vi "update tree.vi"(7 "status type":T1, 8 "error in (no error)":errorcluster, 10 "tag":string, 11 "TreeControl in":refnum<vi>) -> (0 "error out":errorcluster)   [LabVIEW 2016, in "FPGA Addon System Explorer.lvlib"]
uses:
  FPGA Addon System Explorer.lvlib
  reservation type.ctl
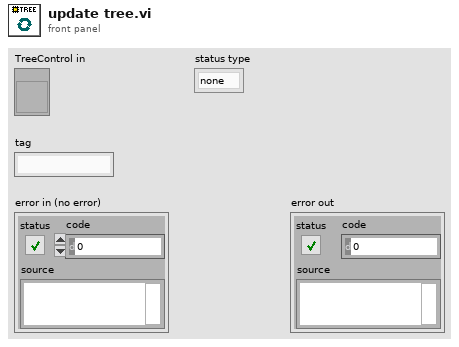
[diagram p1: front panel]
types:
  T1 = typedef "FPGA Addon System Explorer.lvlib/reservation type.ctl" = enum16{"none", "available", "reserved by this", "reserved by other", "incompatible", "parent"}
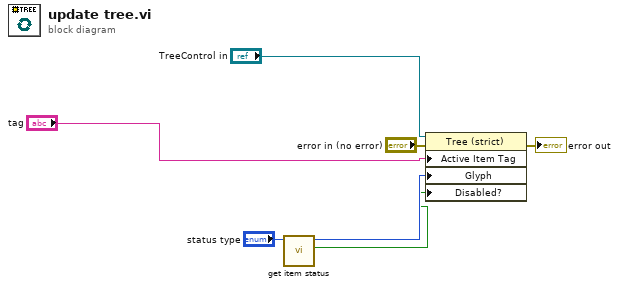
[diagram p0: block diagram]
diagram:
  n1 = call "get item status.vi"("element"="status type") -> ("Disabled?"=w3:bool, "symbol index"=w5:i32)  [unwired: 9 in]
  n2 = property class="Tree (strict)"(reference="TreeControl in", error in="error in (no error)", "Active Item Tag"="tag", "Glyph"=w5, "Disabled?"=w3) -> (error out=→"error out":errorcluster)  [unwired: 1 out]
